vi "Control Panel Values Changed.vi"(8 "error in (no error)":errorcluster, 9 "Old data":variant, 10 "New data":variant, 11 "LakeShore370 in":refnum<class "LakeShore370_device.lvclass">) -> (0 "error out":errorcluster, 3 "LakeShore370 out":refnum<class "LakeShore370_device.lvclass">)   [LabVIEW 2015, in "LakeShore370_device.lvclass"]
uses:
  LakeShore370_device.lvclass
  LakeSore370 Front Panel Data.ctl
  LakeShore370 Heater Ranges.ctl
  Neocera/Neocera Set Point Aproach.ctl
  Instrument/Read VISA Resource.vi
  Instrument/Write VISA Resource.vi
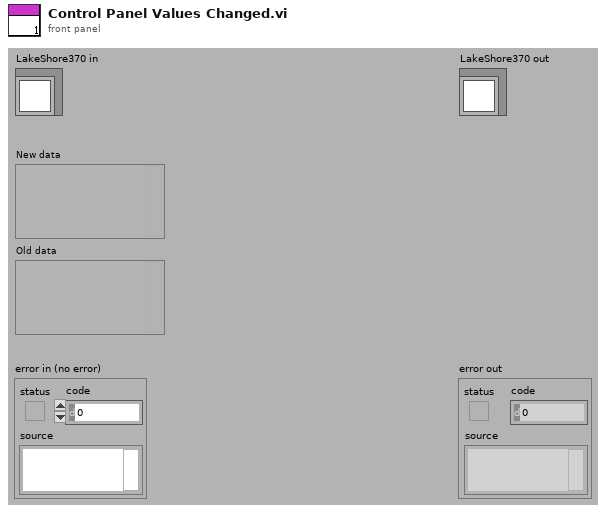
[diagram p1: front panel]
types:
  T1 = typedef "LakeSore370 Front Panel Data.ctl" = cluster{"Channels to scan":i32[], "Scan settling, s":dbl, "Read temperature":bool, "Set point":dbl, "Heater range":T2, "Approach":T3, "Ramp rate, K/min":dbl, "Read heater":bool}
  T2 = typedef "LakeShore370 Heater Ranges.ctl" = enum16{"Off", "31.6uA", "100uA", "316uA", "1mA", "3.16uA", "10mA", "31.6mA", "100mA"}
  T3 = typedef "Neocera Set Point Aproach.ctl" = enum16{"Instant", "Ramp"}
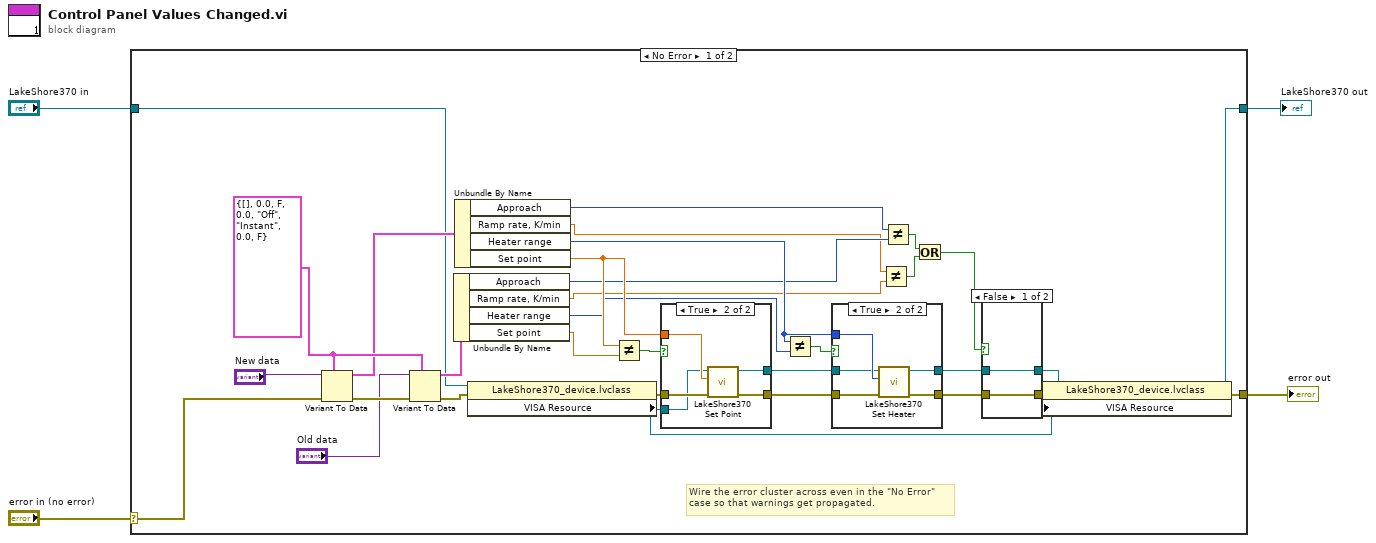
[diagram p0: block diagram]
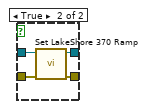
[diagram p2: hidden frame]
diagram:
  n1 = case shown="No Error" "error in (no error)" {
    selector: "error in (no error)" -> [w28 w59]
    tunnel: [w15 w59] -> w3
    tunnel: [w13 w58] -> w1
    tunnel: "LakeShore370 in" -> [w27 w58]
    frame No Error {
      w33 = T1 {"Channels to scan"=[], "Scan settling, s"=0.0, "Read temperature"=FALSE, "Set point"=0.0, "Heater range"=enum."Off", "Approach"=enum."Instant", "Ramp rate, K/min"=0.0, "Read heater"=FALSE} ("Data")
      # "Wire the error cluster across even in the \"No Error\"\ncase so that warnings get propagated."
      n2 = Variant To Data(error in=w28, type=w33, Variant="New data") -> (data=w31:T1, error out=w37:errorcluster)
      n3 = Variant To Data(error in=w37, type=w33, Variant="Old data") -> (data=w36:T1, error out=w25:errorcluster)
      n4 = Unbundle By Name(w36) -> ("Approach"=w10:T3, "Ramp rate, K/min"=w8:dbl, "Heater range"=w19:T2, "Set point"=w35:dbl)
      n5 = Unbundle By Name(w31) -> ("Approach"=w11:T3, "Ramp rate, K/min"=w9:dbl, "Heater range"=w22:T2, "Set point"=w32:dbl)
      n6 = property class="LakeShore370_device.lvclass"(reference=w27, error in=w25) -> (reference out=w14:refnum<class "LakeShore370_device.lvclass">, error out=w24:errorcluster, "VISA Resource"=w26:refnum<visa-resource-name>)
      n7 = Not Equal?(x=w32, y=w35) -> (x != y?=w34:bool)
      n8 = case shown="True" w34 {
        tunnel: w24 -> [w52 w57]
        tunnel: [w52 w54] -> w21
        tunnel: w32 -> [_ w56]
        tunnel: w26 -> [w51 w55]
        tunnel: [w51 w53] -> w20
        frame False {
        }
        frame True {
          n9 = call "LakeShore370 Set Point.vi"("error in (no error)"=w57, "Set Point"=w56, "VISA resource name"=w55) -> ("error out"=w54:errorcluster, "VISA resource name out"=w53:refnum<visa-resource-name>)  [unwired: 7 in]
        }
      }
      n10 = Not Equal?(x=w22, y=w19) -> (x != y?=w23:bool)
      n11 = case shown="True" w23 {
        tunnel: w21 -> [w45 w50]
        tunnel: [w45 w48] -> w18
        tunnel: w22 -> [_ w49]
        tunnel: [w44 w47] -> w16
        tunnel: w20 -> [w44 w46]
        frame False {
        }
        frame True {
          n12 = call "LakeShore370 Set Heater.vi"("error in (no error)"=w50, "Heater range"=w49, "VISA resource name"=w46) -> ("error out"=w48:errorcluster, "VISA resource name out"=w47:refnum<visa-resource-name>)  [unwired: 7 in]
        }
      }
      n13 = Not Equal?(x=w9, y=w8) -> (x != y?=w6:bool)
      n14 = Not Equal?(x=w11, y=w10) -> (x != y?=w7:bool)
      n15 = Or(x=w7, y=w6) -> (x .or. y?=w5:bool)
      n16 = case shown="False" w5 {
        tunnel: w18 -> [w38 w43]
        tunnel: [w38 w42] -> w17
        tunnel: w16 -> [w39 w41]
        tunnel: [w39 w40] -> w12
        frame False {
        }
        frame True {
          n17 = call "Set LakeShore 370 Ramp.vi"("error in (no error)"=w43, "VISA resource name"=w41) -> ("error out"=w42:errorcluster, "VISA resource name out"=w40:refnum<visa-resource-name>)  [unwired: 8 in]
        }
      }
      n18 = property class="LakeShore370_device.lvclass"(reference=w14, error in=w17, "VISA Resource"=w12) -> (reference out=w13:refnum<class "LakeShore370_device.lvclass">, error out=w15:errorcluster)
    }
    frame Error {
    }
  }
  "error out" <- w3
  "LakeShore370 out" <- w1
